vi "EminemGlobals.vi"() -> ()   [LabVIEW 2023]
uses:
  EminemStatesEnum.ctl
panel:
  out "BotShooterSpeedSP":dbl
  out "TopShooterSpeedSP":dbl
  out "Tune_Kizone":dbl=350.0
  out "Tune_Ki":dbl=3.0
  out "Tune_Kp":dbl=0.7
  out "Tune_TopKn":dbl=0.000177245949924187
  out "Tune_BotKn":dbl=0.000177245949924187
  out "Tune_BotKv":dbl=0.000174
  out "Tune_TopKs":dbl=0.018313253
  out "Tune_BotKs":dbl=0.018313253
  out "Tune_TopKv":dbl=0.000174
  out "Tune_FeedAmpMtrDmd":dbl=0.3
  out "Tune_FeedShootMtrDmd":dbl=0.95
  out "Tune_ShootSpeedDmd":dbl=2000.0
  out "Tune_BotAmpSpeedDmd":dbl
  out "Tune_TopAmpSpeedDmd":dbl=-300.0
  out "ShootRevUp":bool
  out "FeedMtrSpeed":dbl
  out "ShooterSpeedRPM_FB":dbl=4000.0
  out "BotShooterMotorOutput":dbl
  out "TopShooterMotorOutput":dbl
  out "BotShooterFilteredSpeed":dbl
  out "BotShooterSpeed":dbl
  out "TopShooterFilteredSpeed":dbl
  out "TopShooterSpeed":dbl
  out "MNM_State":T1=enum."13-AmpDone"
  out "BotAtSpeed":bool
  out "TopAtSpeed":bool
  out "FeedMtrOutput":dbl=0.5
  out "ShooterSpeedRPM":dbl=4000.0
  out "ReadyForCommand":bool
  # "Speed / Motor Out Setpoints"
  # "Calc"
  # "Tuning"
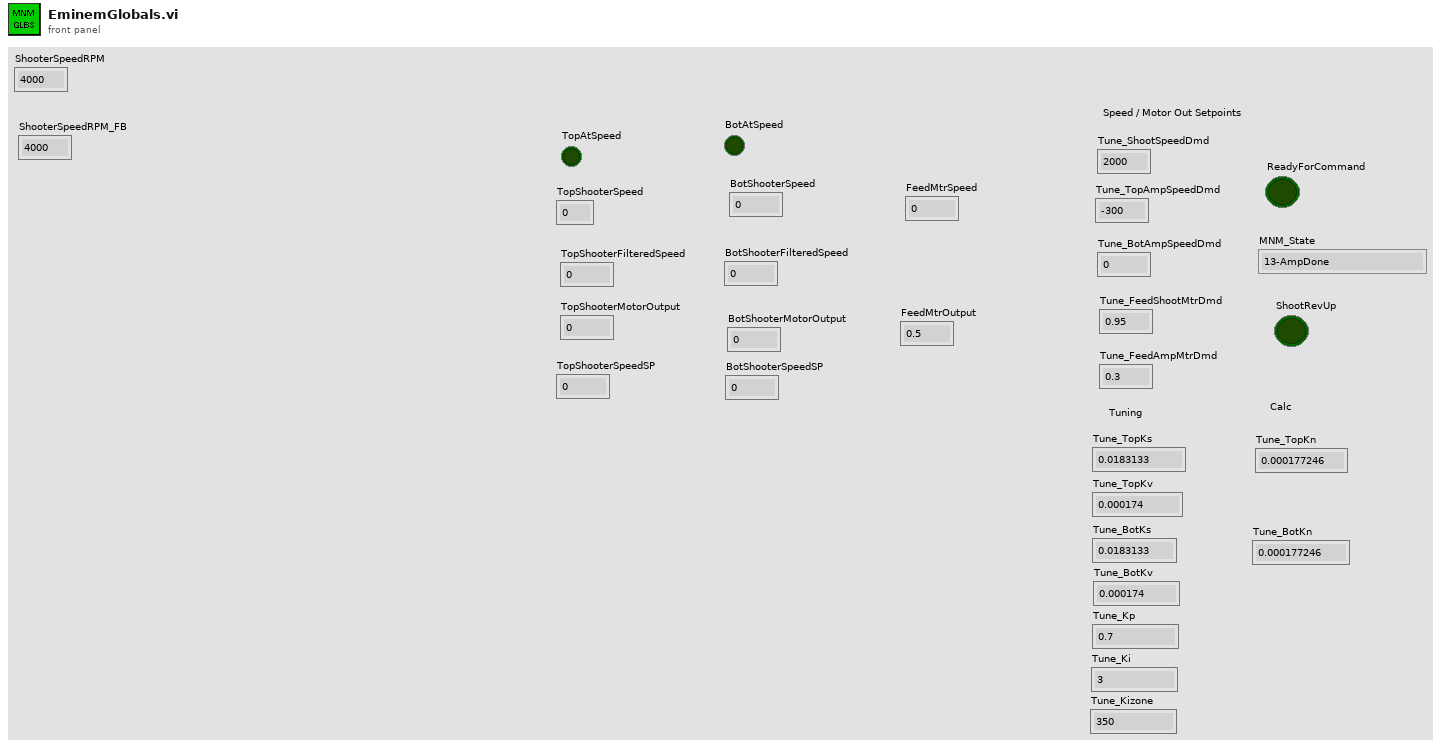
[diagram p1: front panel]
types:
  T1 = typedef "EminemStatesEnum.ctl" = enum16{"0-Init", "1-WaitForCmd", "2-Cancel", "3-ShootStart", "4-ShootRev", "5-RevUpStart", "6-ShootStartFeed&Timer", "7-ShootTimerOrSensorDone", "8-ShootDone", "9-AmpStart", "10-AmpUpToSpd?", "11-AmpStartFeed&Timer", "12-AmpTimerOrSensorDone", "13-AmpDone", "14-RevUpGetCmd"}
diagram:
